vi "Write currentState.vi"(8 "error in (no error)":errorcluster, 10 "Enum":T1, 11 "WaitPassTactic in":refnum<class "WaitPassTactic.lvclass">) -> (0 "error out":errorcluster, 3 "WaitPassTactic out":refnum<class "WaitPassTactic.lvclass">)   [LabVIEW 2023, in "WaitPassTactic.lvclass"]
uses:
  WaitPassTactic.lvclass
  WaitPassTactic_states_class/WaitPassTactic_states.ctl
  WaitPassTactic.lvclass/WaitPassTactic.ctl
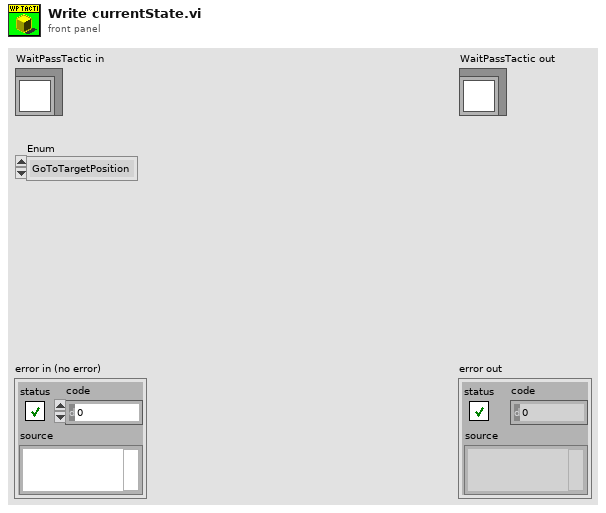
[diagram p1: front panel]
types:
  T1 = typedef "WaitPassTactic.lvclass/WaitPassTactic_states.ctl" = enum16{"GoToTargetPosition", "InterceptBall", "Exit"}
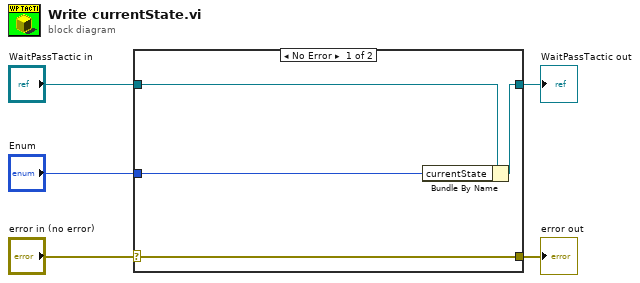
[diagram p0: block diagram]
diagram:
  n1 = case shown="No Error" "error in (no error)" {
    selector: "error in (no error)" -> [w9 w10]
    tunnel: [w9 w10] -> w4
    tunnel: [w7 w11] -> w2
    tunnel: "WaitPassTactic in" -> [w8 w11]
    tunnel: "Enum" -> [w6 _]
    frame No Error {
      n2 = Bundle By Name(cluster=w8, "currentState"=w6) -> (w7:refnum<class "WaitPassTactic.lvclass">)
    }
    frame Error {
    }
  }
  "error out" <- w4
  "WaitPassTactic out" <- w2
